vi "MDTFlavorToTypeEnum.vi"(11 "MDTFlavor":i16) -> (3 "Data Type":T1=enum."Digital Waveform")   [LabVIEW 2020, in "NI_Data Type.lvlib"]
doc: "Convert MDTFlavor value to Data Type enum."
uses:
  <vilib>/Utility/Data Type/NI_Data Type.lvlib
  <vilib>/Utility/Data Type/Type Definitions/Data Type.ctl
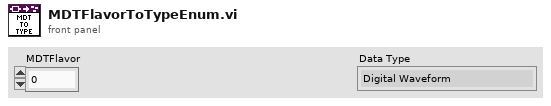
[diagram p1: front panel]
types:
  T1 = typedef "NI_Data Type.lvlib/Data Type.ctl" = enum8{"Invalid Type", "Void", "I8", "I16", "I32", "I64", "U8", "U16", "U32", "U64", "Single Float", "Double Float", "Extended Float", "Single Complex", "Double Complex", "Extended Complex", "Enum U8", "Enum U16", "Enum U32", "Enum U64", "Single Float With Unit", "Double Float With Unit", "Extended Float With Unit", "Single Complex with Unit", "Double Complex with Unit", "Extended Complex with Unit", "Boolean", "String", "Path", "Picture", "Tag", "Array", "Cluster", "Variant", "LV Variant", "Waveform", "Timestamp", "Digital Waveform", "Digital Data", "ExpressData", "Refnum", "External Data", "VI", "Poly VI", "LabVIEW Class Instance", "Fixed Point", "Set Collection", "Map Collection"}
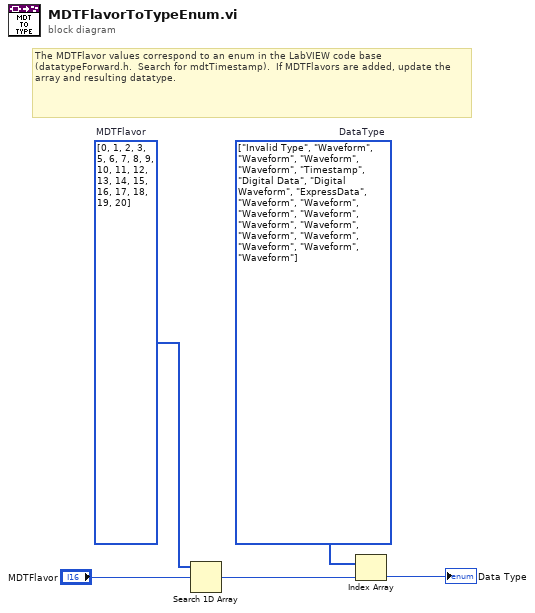
[diagram p0: block diagram]
diagram:
  w1 = T1[] [enum."Invalid Type", enum."Waveform", enum."Waveform", enum."Waveform", enum."Waveform", enum."Timestamp", enum."Digital Data", enum."Digital Waveform", enum."ExpressData", enum."Waveform", enum."Waveform", enum."Waveform", enum."Waveform", enum."Waveform", enum."Waveform", enum."Waveform", enum."Waveform", enum."Waveform", enum."Waveform", enum."Waveform"] items=["Invalid Type", "Void", "I8", "I16", "I32", "I64", "U8", "U16", "U32", "U64", "Single Float", "Double Float", "Extended Float", "Single Complex", "Double Complex", "Extended Complex", "Enum U8", "Enum U16", "Enum U32", "Enum U64", "Single Float With Unit", "Double Float With Unit", "Extended Float With Unit", "Single Complex with Unit", "Double Complex with Unit", "Extended Complex with Unit", "Boolean", "String", "Path", "Picture", "Tag", "Array", "Cluster", "Variant", "LV Variant", "Waveform", "Timestamp", "Digital Waveform", "Digital Data", "ExpressData", "Refnum", "External Data", "VI", "Poly VI", "LabVIEW Class Instance", "Fixed Point", "Set Collection", "Map Collection"]  # DataType
  w5 = i16[] [0, 1, 2, 3, 5, 6, 7, 8, 9, 10, 11, 12, 13, 14, 15, 16, 17, 18, 19, 20]  # MDTFlavor
  # "The MDTFlavor values correspond to an enum in the LabVIEW code base (datatypeForward.h.  Search for mdtTimestamp).  If MDTFlavors are added, update the array and resulting datatype."
  n1 = Search 1D Array(1D array=w5, element="MDTFlavor") -> (index of element=w3:i32)  [unwired: 1 in]
  n2 = Index Array(array=w1, index=w3) -> (element=→"Data Type":T1)
